vi "Query XML Document for a Single Node.vi"(8 "error in (no error)":errorcluster, 10 "XML document":string="<?xml version=\"1.0\" encoding=\"ISO-8859-1\"?>\n<bookstore>\n<book ISBN=\"978-0545128285\">\n  <title lang=\"en\">The Tales of Beedle the Bard</title>\n  <author>J. K. Rowling</author>\n  <year>2008</year>\n  <price>12.99</price>\n</book>\n<book ISBN=\"978-0316160209\">\n  <title lang=\"en\">Eclipse</title>\n  <author>Stephenie Meyer</author>\n  <year>2007</year>\n  <price>19.99</price>\n</book>\n<book ISBN=\"978-0316067928\">\n  <title lang=\"en\">Breaking Dawn</title>\n  <author>Stephenie Meyer</author>\n  <year>2008</year>\n  <price>22.99</price>\n</book>\n<book ISBN=\"978-0316017923\">\n  <title lang=\"en\">Outliers: The Story of Success</title>\n  <author>Malcolm Gladwell</author>\n  <year>2008</year>\n  <price>27.99</price>\n</book>\n<book ISBN=\"978-0596007645\">\n  <title lang=\"en\">XML in a Nutshell</title>\n  <author>Elliotte Rusty Harold</author>\n  <author>W. Scott Means</author>\n  <year>2004</year>\n  <price>39.95</price>\n</book>\n</bookstore>", 11 "XPath expression":string="/bookstore/book/title") -> (0 "error out":errorcluster, 2 "match found?":bool, 3 "Result XML":string)   [LabVIEW 2017]
doc: "This example demonstrates how to query an XML document by using an XPath expression and returns the first node that matches the XPath expression."
uses:
  <vilib>/xml/Load XML String.vi
  <vilib>/xml/Close Reference(Node).vi
  <vilib>/xml/NI_XML.lvlib
  <resource>/objmgr/DOMUserDefRef.rc
panel:
  # "This example demonstrates how to query an XML document by using an XPath expression and returns the first node that \nmatches the XPath expression."
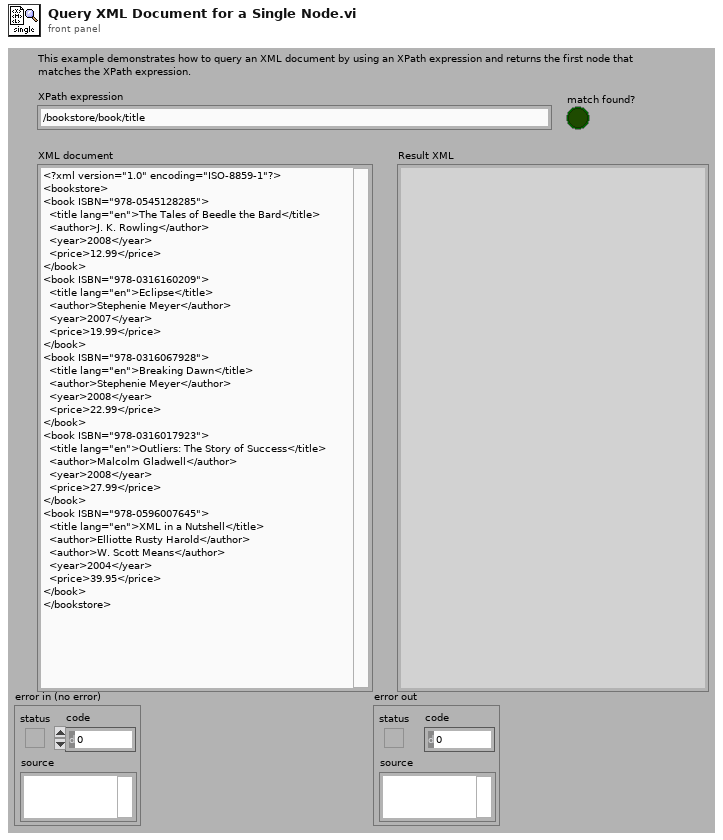
[diagram p1: front panel]
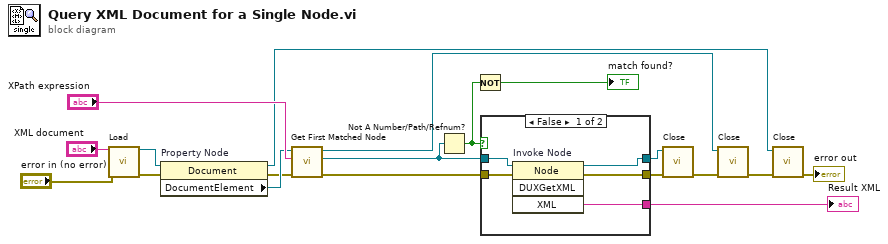
[diagram p0: block diagram]
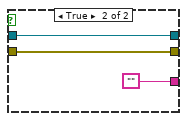
[diagram p2: hidden frame]
diagram:
  n1 = call-poly <vilib>:"Load.vi"("XML string"="XML document", "error in (no error)"="error in (no error)") -> ("DOM document out"=w12:refnum<k20>, "error out"=w10:errorcluster)  [unwired: 12 out]
  n2 = property on="Property Node" class="Document"(reference=w12, error in=w10) -> (reference out=w7:refnum<k20>, error out=w9:errorcluster, "DocumentElement"=w11:refnum<k20>)
  n3 = call <vilib>:"Get First Matched Node.vi"("error in (no error)"=w9, "XPath expression"="XPath expression", "node in"=w11) -> ("error out"=w17:errorcluster, "node result"=w5:refnum<k20>, "node out"=w13:refnum<k20>)  [unwired: 6 out]
  n4 = Not A Number/Path/Refnum?(number/path/refnum=w5) -> (NaN/Path/Refnum?=w3:bool)
  n5 = Not(x=w3) -> (.not. x?=→"match found?":bool)
  n6 = case shown="False" w3 {
    tunnel: w17 -> [w24 w27]
    tunnel: [w23 w26] -> w15
    tunnel: [w22 w27] -> w14
    tunnel: [w21 ""] -> w6
    tunnel: w5 -> [w20 w26]
    frame False {
      n7 = invoke on="Invoke Node" class="Node" method="DUXGetXML"(reference=w20, error in=w24) -> (reference out=w23:refnum<k20>, error out=w22:errorcluster, "XML"=w21:string)  [unwired: 2 in, 1 out]
    }
    frame True {
    }
  }
  "Result XML" <- w6
  n8 = call-poly <vilib>:"Close.vi"("error in (no error)"=w14, "node"=w15) -> ("error out"=w16:errorcluster)  [unwired: 7 out]
  n9 = call-poly <vilib>:"Close.vi"("error in (no error)"=w16, "node"=w13) -> ("error out"=w8:errorcluster)  [unwired: 7 out]
  n10 = call-poly <vilib>:"Close.vi"("error in (no error)"=w8, "node"=w7) -> ("error out"=→"error out":errorcluster)  [unwired: 7 out]
